vi "Get Direction.vi"(9 "Column":i32, 10 "Row":i32, 11 "AntFarm_MB":refnum<class "AntFarm_MB.lvclass">) -> (2 "Direction Out":T1, 3 "AntFarm_MB Out":refnum<class "AntFarm_MB.lvclass">)   [LabVIEW 2017, in "AntFarm_MB.lvclass"]
uses:
  AntFarm_MB.lvclass
  Type Defs/Direction Enum.ctl
  TypeDefs/Cluster_Ant Farm Global Data.ctl
  AntFarm_MB.lvclass/AntFarm_MB.ctl
  Type Defs/SB Type Defs.lvlib
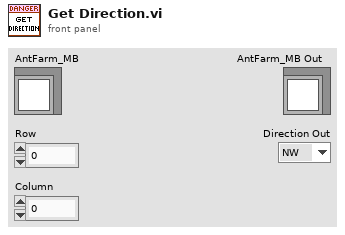
[diagram p1: front panel]
types:
  T1 = typedef "SB Type Defs.lvlib/Direction Enum.ctl" = enum16{"NW", "N", "NE", "E", "SE", "S", "SW", "W"}
  T2 = typedef "Cluster_Ant Farm Global Data.ctl" = cluster{"Move Map":i32[][], "Danger Map":i32[][], "Attack Rows":i32[], "Attack Columns":i32[], "Square count":i32, "Last Round":i32, "Danger Threshold":i32}
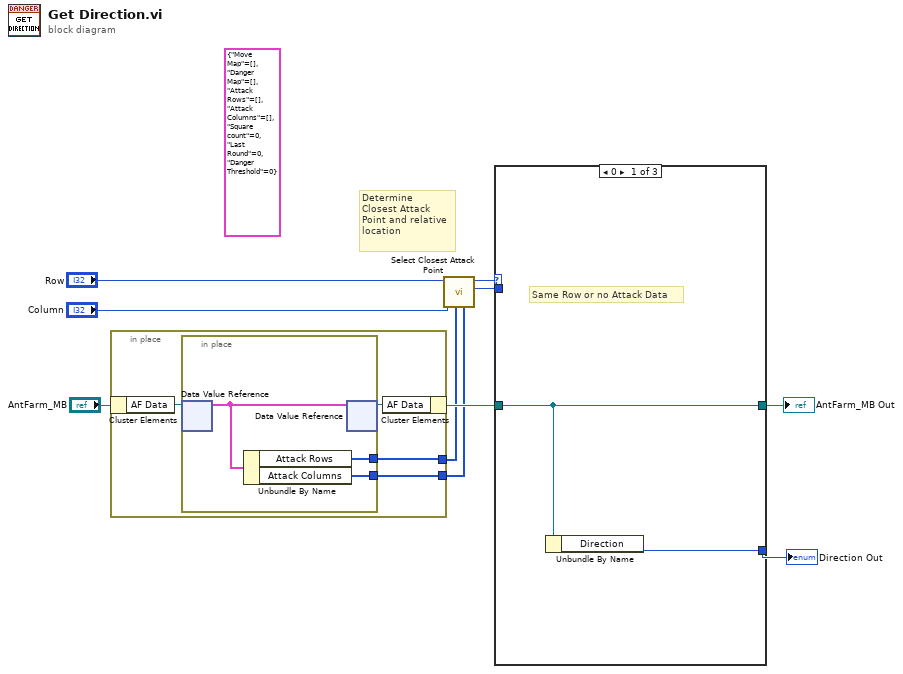
[diagram p0: block diagram]
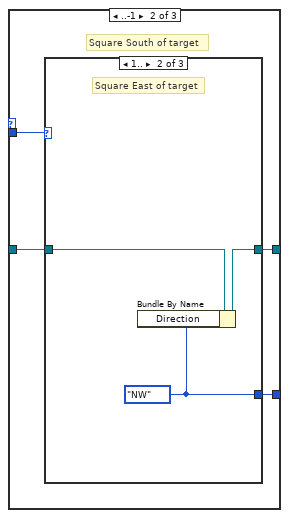
[diagram p2: hidden frame]
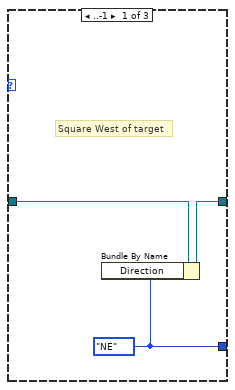
[diagram p3: hidden frame]
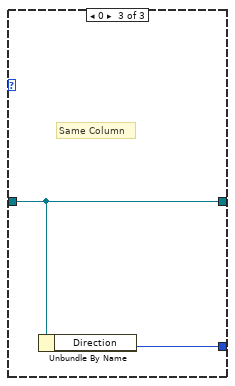
[diagram p4: hidden frame]
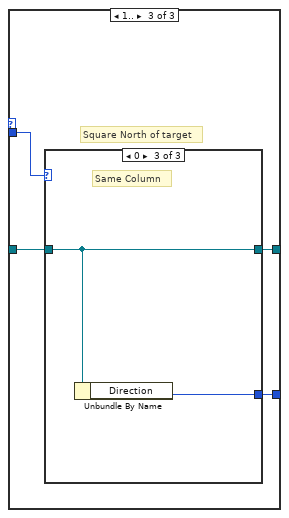
[diagram p5: hidden frame]
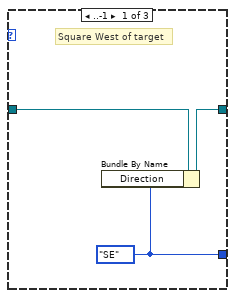
[diagram p6: hidden frame]
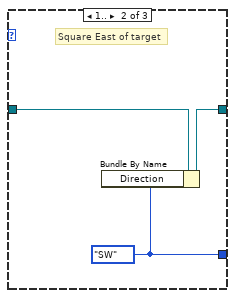
[diagram p7: hidden frame]
diagram:
  (unwired) T2 {"Move Map"=[], "Danger Map"=[], "Attack Rows"=[], "Attack Columns"=[], "Square count"=0, "Last Round"=0, "Danger Threshold"=0} ("data value")
  # "Determine\nClosest Attack\nPoint and relative\nlocation"
  n1 = in-place {
    in-place-border: [w12] -> w5
    in-place-border: [w11] -> w8
    n2 = in-place-cluster #1("AntFarm_MB") -> ("AF Data"=w14:refnum<data-value>)
    n3 = in-place {
      in-place-border: [w16] -> w12
      in-place-border: [w15] -> w11
      n4 = in-place-dvr #2(w14) -> (w17:T2)  [unwired: 1 out]
      n5 = Unbundle By Name(w17) -> ("Attack Rows"=w16:i32[], "Attack Columns"=w15:i32[])
      n6 = in-place-dvr #2(w17) -> (w13:refnum<data-value>)  [unwired: 1 out]
    }
    n7 = in-place-cluster #1("AF Data"=w13) -> (w9:refnum<class "AntFarm_MB.lvclass">)
  }
  n8 = call "Select Closest Attack Point.vi"("Attack Columns"=w8, "Attack Rows"=w5, "Column"="Column", "Row"="Row") -> ("Relative Column Location"=w3:i32, "Relative  Row Location"=w4:i32)  [unwired: 6 in]
  n9 = case shown="0" w4 {
    tunnel: w3 -> [_ w23 w35]
    tunnel: [w18 w22 w34] -> w7
    tunnel: w9 -> [w19 w21 w33]
    tunnel: [w19 w20 w32] -> w6
    frame 0 {
      # "Same Row or no Attack Data"
      n10 = Unbundle By Name(w19) -> ("Direction"=w18:T1)
    }
    frame ..-1 {
      # "Square South of target"
      n11 = case shown="1.." w23 {
        tunnel: [w24 w27 w30] -> w22
        tunnel: w21 -> [w26 w29 w31]
        tunnel: [w25 w28 w31] -> w20
        frame ..-1 {
          w24 = Direction_Enum."NE" ("Direction")
          # "Square West of target"
          n12 = Bundle By Name(cluster=w26, "Direction"=w24) -> (w25:refnum<class "AntFarm_MB.lvclass">)
        }
        frame 1.. {
          w27 = Direction_Enum."NW" ("Direction")
          # "Square East of target"
          n13 = Bundle By Name(cluster=w29, "Direction"=w27) -> (w28:refnum<class "AntFarm_MB.lvclass">)
        }
        frame 0 {
          # "Same Column"
          n14 = Unbundle By Name(w31) -> ("Direction"=w30:T1)
        }
      }
    }
    frame 1.. {
      # "Square North of target"
      n15 = case shown="0" w35 {
        tunnel: [w36 w39 w42] -> w34
        tunnel: w33 -> [w38 w41 w43]
        tunnel: [w37 w40 w43] -> w32
        frame ..-1 {
          w36 = Direction_Enum."SE" ("Direction")
          # "Square West of target"
          n16 = Bundle By Name(cluster=w38, "Direction"=w36) -> (w37:refnum<class "AntFarm_MB.lvclass">)
        }
        frame 1.. {
          w39 = Direction_Enum."SW" ("Direction")
          # "Square East of target"
          n17 = Bundle By Name(cluster=w41, "Direction"=w39) -> (w40:refnum<class "AntFarm_MB.lvclass">)
        }
        frame 0 {
          # "Same Column"
          n18 = Unbundle By Name(w43) -> ("Direction"=w42:T1)
        }
      }
    }
  }
  "AntFarm_MB Out" <- w6
  "Direction Out" <- w7
